vi "GetControlValue_Variant.vi"(8 "error in (no error)":errorcluster, 9 "Expected Data Type":variant, 10 "Control Label":string, 11 "CtlLookup In":T1) -> (0 "error out":errorcluster, 2 "Value":variant, 3 "CtlLookup In":T1)   [LabVIEW 2020, in "CtlReferences.lvlib" / "CtlReferences.lvclass"]
doc: "This VI uses the GetControlByReference to get the specified control as a variant"
uses:
  CtlReferences.lvclass
  TypeDefs/CtlLookup.ctl
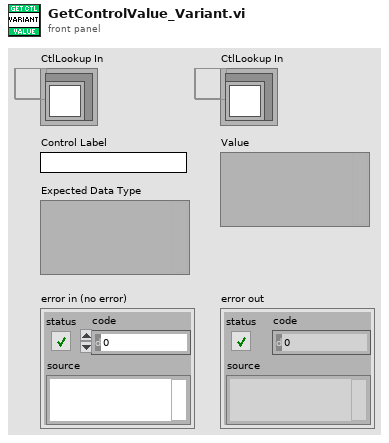
[diagram p1: front panel]
types:
  T1 = typedef "CtlReferences.lvlib/CtlReferences.lvclass/CtlLookup.ctl" = refnum<data-value>
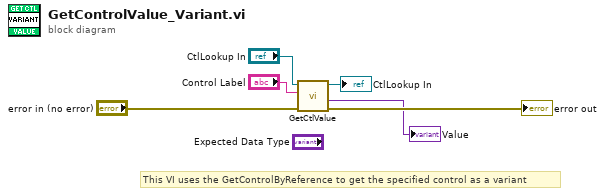
[diagram p0: block diagram]
diagram:
  # "This VI uses the GetControlByReference to get the specified control as a variant"
  n1 = call "GetCtlValue.vi"("Error in"="error in (no error)", "CtlName In"="Control Label", "CtlLookup In"="CtlLookup In") -> ("error out"=→"error out":errorcluster, "Value"=→"Value":variant, "CtlLookup Out"=→"CtlLookup In":T1)  [unwired: 6 in]
